vi "Bundle Current Actor VI Ref.vi"(8 "error in (no error)":errorcluster, 10 "This VI":refnum<vi>, 11 "UI ActorTop in":refnum<class "UIActorTop.lvclass">) -> (0 "error out":errorcluster, 2 "Controls Name List":string, 3 "UI ActorTop out":refnum<class "UIActorTop.lvclass">)   [LabVIEW 2021, in "AbstractActorTemplate.lvlib" / "UIActorTop.lvclass"]
uses:
  <userlib>/John_Lib/AbstractActorTemplate/AbstractActorTemplate/UIActorTop.lvclass
  <userlib>/John_Lib/AbstractActorTemplate/AbstractActorTemplate/UIActorTop.lvclass/UIActorTop.ctl
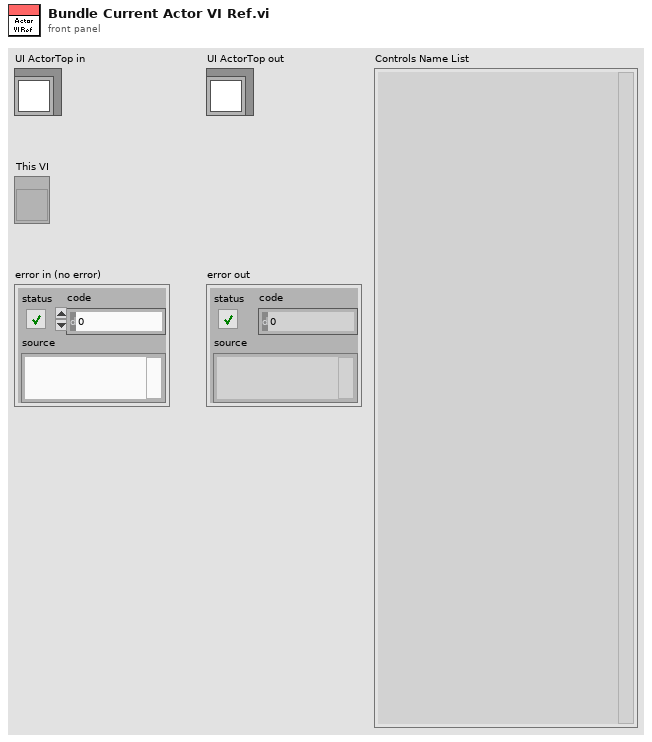
[diagram p1: front panel]
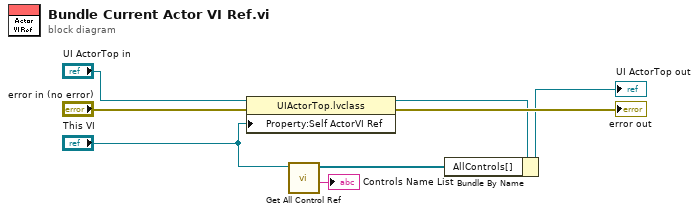
[diagram p0: block diagram]
diagram:
  n1 = property class="UIActorTop.lvclass"(reference="UI ActorTop in", error in="error in (no error)", "Property:Self ActorVI Ref"="This VI") -> (reference out=w5:refnum<class "UIActorTop.lvclass">, error out=→"error out":errorcluster)
  n2 = call <userlib>:"Get All Control Ref.vi"("reference"="This VI") -> ("Controls Name List"=→"Controls Name List":string, "Controls[]"=w2:refnum<vi>[])  [unwired: 8 in, 1 out]
  n3 = Bundle By Name(cluster=w5, "AllControls[]"=w2) -> (→"UI ActorTop out":refnum<class "UIActorTop.lvclass">)
